vi "Operate.vi"(8 "error in (no error)":errorcluster, 11 "Add in":refnum<class "Add.lvclass">) -> (0 "error out":errorcluster, 3 "Add out":refnum<class "Add.lvclass">)   [LabVIEW 2020, in "Add.lvclass"]
doc: "This method is a child method which is used to perform the add operation"
uses:
  Add.lvclass
  C:/Users/khishore.kumar/Khishore/labview_tips_2024/src/Assignment 24/Math Operations/Math Operations.lvclass
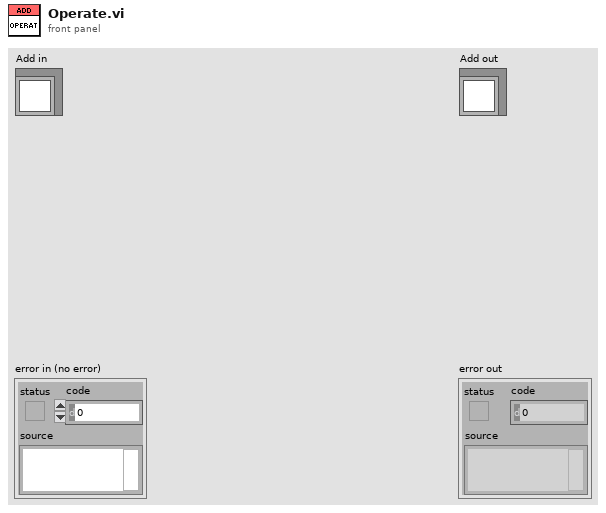
[diagram p1: front panel]
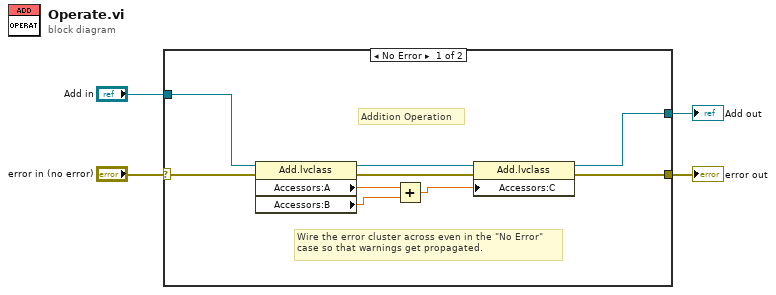
[diagram p0: block diagram]
diagram:
  n1 = case shown="No Error" "error in (no error)" {
    selector: "error in (no error)" -> [w13 w15]
    tunnel: [w5 w15] -> w3
    tunnel: [w6 w14] -> w1
    tunnel: "Add in" -> [w12 w14]
    frame No Error {
      # "Addition Operation"
      # "Wire the error cluster across even in the \"No Error\"\ncase so that warnings get propagated."
      n2 = property class="Add.lvclass"(reference=w12, error in=w13) -> (reference out=w7:refnum<class "Add.lvclass">, error out=w8:errorcluster, "Accessors:A"=w11:dbl, "Accessors:B"=w10:dbl)
      n3 = Add(x=w11, y=w10) -> (x+y=w9:dbl)
      n4 = property class="Add.lvclass"(reference=w7, error in=w8, "Accessors:C"=w9) -> (reference out=w6:refnum<class "Add.lvclass">, error out=w5:errorcluster)
    }
    frame Error {
    }
  }
  "error out" <- w3
  "Add out" <- w1
